vi "Assertion Failure Message.vi"() -> ()   [LabVIEW 2017, in "Assertions.Tests.lvlib" / "Assert Not Equal.lvlib"]
uses:
  Assert Not Equal.lvlib
  src/Transparent Assertions/Constraints/IsEqual/IsEqual.lvclass
  C:/Users/pasca/Projects/Home/TransparentAssertions/src/Transparent Assertions/Constraints/Constraint/Constraint.lvclass
  src/Transparent Assertions/Constraints/IsEqual/Create.vi
  src/Transparent Assertions/Constraints/LogicalNot/LogicalNot.lvclass
  src/Transparent Assertions/Constraints/UnaryOperator/UnaryOperator.lvclass
  src/Transparent Assertions/Assertions/Assertions.lvlib
panel:
  out "error out":errorcluster
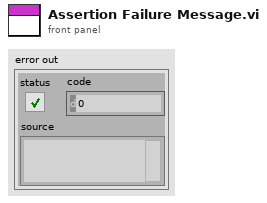
[diagram p1: front panel]
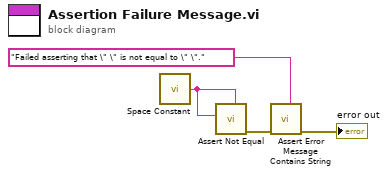
[diagram p0: block diagram]
diagram:
  n1 = call <vilib>:"Space Constant.vi"() -> ("String"=w1:string)
  n2 = call "Assert Not Equal.vi"("Expected"=w1, "Actual"=w1) -> ("error out"=w4:errorcluster)  [unwired: 9 in]
  n3 = call "Assert Error Message Contains String.vi"("Expected"="Failed asserting that \" \" is not equal to \" \"." ("y"), "error in (no error)"=w4) -> ("error out"=→"error out":errorcluster)  [unwired: 9 in]
